vi "Create Datafile.vi"(0 "object in":refnum<class "SaveData.lvclass">, 2 "Path":path, 5 "error in (no error)":errorcluster) -> (14 "object out":refnum<class "SaveData.lvclass">, 19 "error out":errorcluster)   [LabVIEW 2023, in "SaveData.lvclass"]
uses:
  SaveData.lvclass
  SaveData.lvclass/SaveData.ctl
  <vilib>/Utility/NIReport.llb/NI_report.lvclass
  <vilib>/Utility/NIReport.llb/Report Type.ctl
  <vilib>/Utility/NIReport.llb/NI_ReportGenerationCore.lvlib
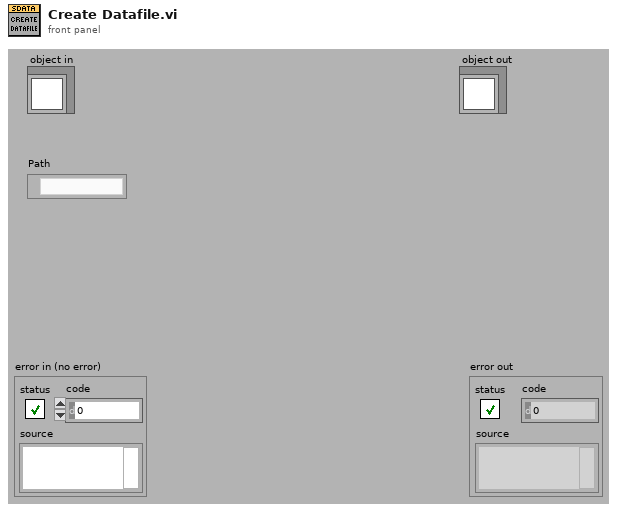
[diagram p1: front panel]
types:
  T1 = typedef "NI_ReportGenerationCore.lvlib/Report Type.ctl" = enum16{"HTML", "Word", "Excel"}
  T2 = enum16{"open", "replace", "create", "open or create", "replace or create", "replace or create with confirmation"}
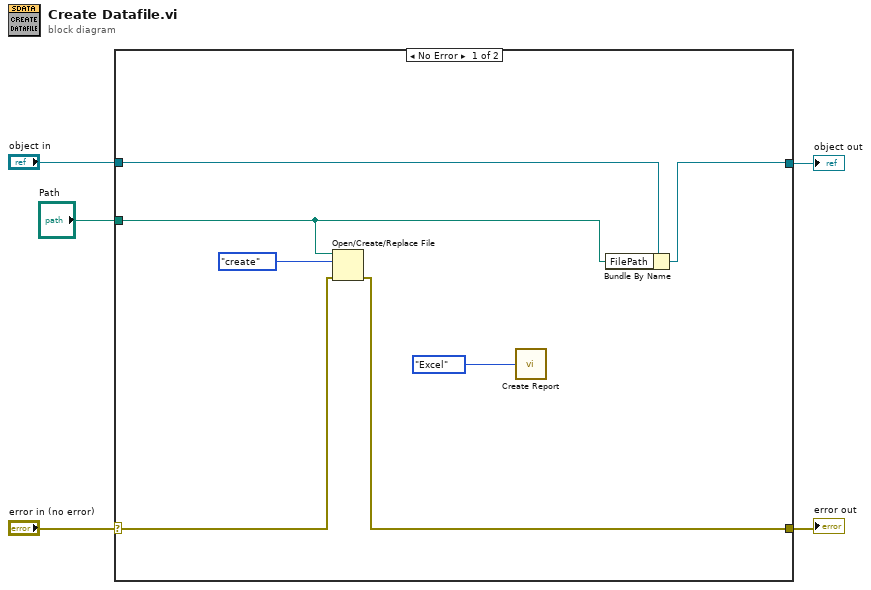
[diagram p0: block diagram]
diagram:
  n1 = case shown="No Error" "error in (no error)" {
    selector: "error in (no error)" -> [w10 w14]
    tunnel: [w11 w14] -> w4
    tunnel: [w9 w13] -> w3
    tunnel: "object in" -> [w8 w13]
    tunnel: "Path" -> [w7 _]
    frame No Error {
      n2 = Open/Create/Replace File(file path (use dialog)=w7, error in=w10, operation (0:open)=T2."create") -> (error out=w11:errorcluster)  [unwired: 3 in, 2 out]
      n3 = call <vilib>:"Create Report.vi"("report type"=Report_Type."Excel") -> ()  [unwired: 13 in, 2 out]
      n4 = Bundle By Name(cluster=w8, "FilePath"=w7) -> (w9:refnum<class "SaveData.lvclass">)
    }
    frame Error {
    }
  }
  "error out" <- w4
  "object out" <- w3
